vi "process_reaction_methodr.vi"() -> ()   [LabVIEW 2021]
uses:
  <vilib>/Analysis/NI_AALPro.lvlib
panel:
  out "appended array":dbl[][](array[numeric])=[[0.0, 0.0], [0.4, 0.01], [0.8, 0.07], [1.2, 0.17], [1.6, 0.31], [2.0, 0.46], [2.4, 0.62], [2.8, 0.76], [3.2, 0.88], [3.6, 0.99], [4.0, 1.09], [4.4, 1.16], [4.8, 1.22], [5.2, 1.27], [5.6, 1.31], [6.0, 1.34], [6.4, 1.36], [6.8, 1.38], [7.2, 1.39], [7.6, 1.4], [8.0, 1.412], [8.4, 1.41], [8.8, 1.427], [9.6, 1.42], [10.0, 1.42]]
  in  "Values for output y":dbl[](array[numeric])=[0.0, 0.01, 0.07, 0.17, 0.31, 0.46, 0.62, 0.76, 0.88, 0.99, 1.09, 1.16, 1.22, 1.27, 1.31, 1.34, 1.36, 1.38, 1.39, 1.4, 1.412, 1.41, 1.427, 1.42, 1.42]
  in  "values for time t":dbl[](array[numeric])=[0.0, 0.4, 0.8, 1.2, 1.6, 2.0, 2.4, 2.8, 3.2, 3.6, 4.0, 4.4, 4.8, 5.2, 5.6, 6.0, 6.4, 6.8, 7.2, 7.6, 8.0, 8.4, 8.8, 9.6, 10.0]
  out "L":dbl=0.8000000000000003
  out "T":dbl=3.664516129032257
  out "K":dbl=1.42
  out "max index(es)":i32=5
  out "max dy/dt":dbl=0.38750000000000007
  out "output array 2":dbl[](array[numeric])=[0.0, 0.4, 0.8, 1.2, 1.6, 2.0, 2.4, 2.8, 3.2, 3.6, 4.0, 4.4, 4.8, 5.2, 5.6, 6.0, 6.4, 6.8, 7.2, 7.6, 8.0, 8.4, 8.8, 9.6, 10.0]
  out "output array":dbl[](array[numeric])=[0.0, 0.01, 0.07, 0.17, 0.31, 0.46, 0.62, 0.76, 0.88, 0.99, 1.09, 1.16, 1.22, 1.27, 1.31, 1.34, 1.36, 1.38, 1.39, 1.4, 1.412, 1.41, 1.427, 1.42, 1.42]
  in  "U":dbl=1.0
  out "Delta_Y":dbl=1.42
  out "size(s)":i32[](array[numeric])=[25, 2]
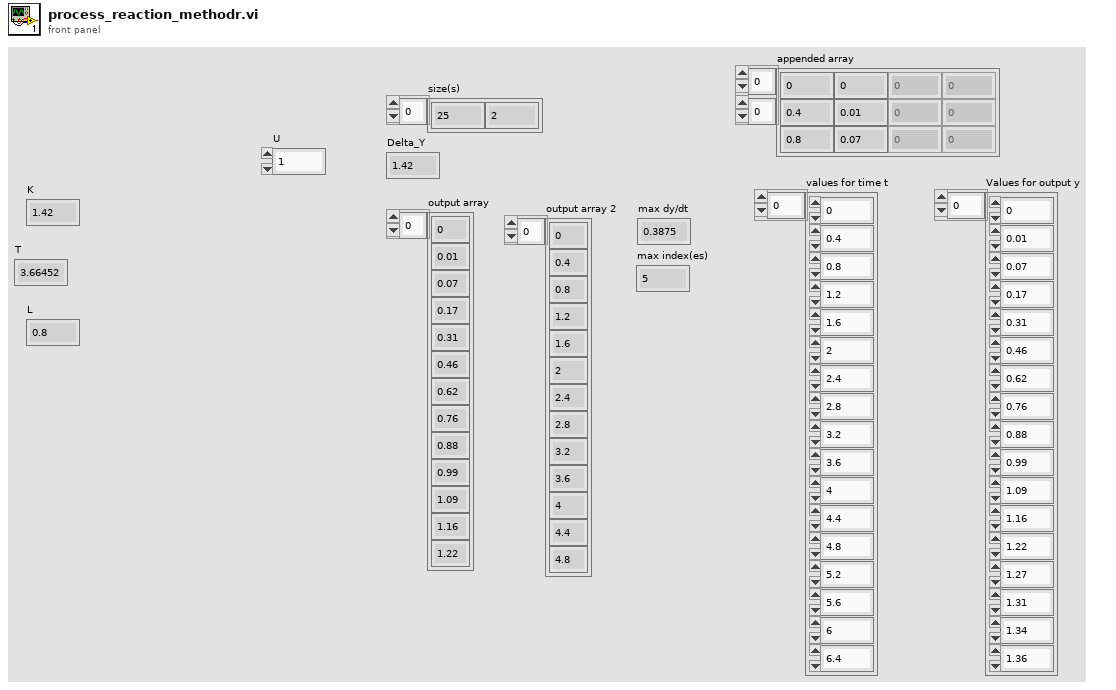
[diagram p1: front panel]
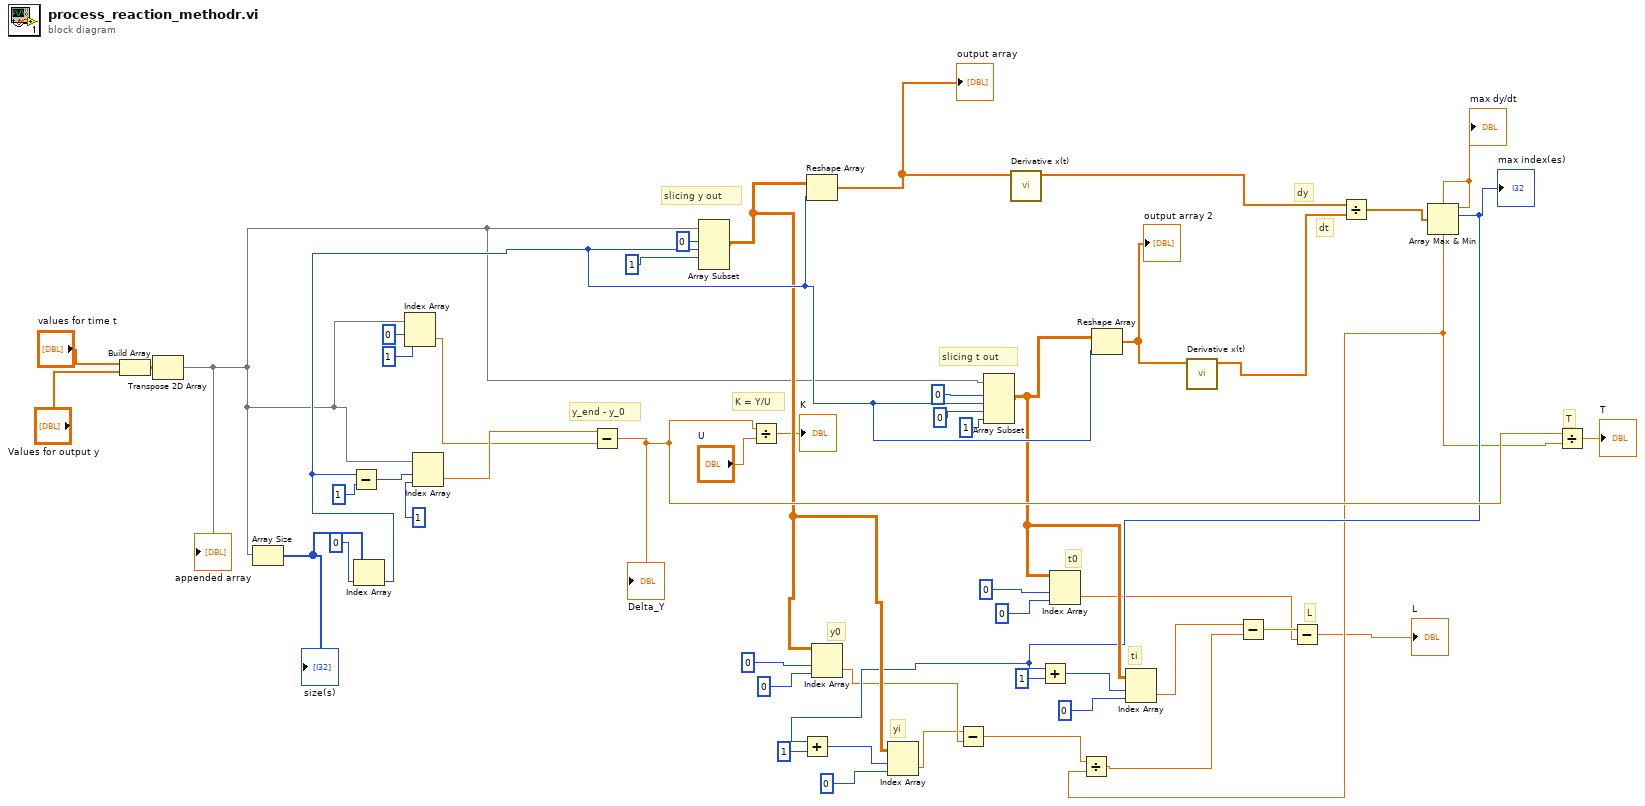
[diagram p0: block diagram]
diagram:
  # "L"
  # "yi"
  # "y0"
  # "ti"
  # "t0"
  # "T"
  # "dt"
  # "dy"
  # "slicing t out"
  # "slicing y out"
  # "K = Y/U"
  # "y_end - y_0"
  n1 = Build Array("values for time t", "Values for output y") -> (w2:dbl[][])
  n2 = Transpose 2D Array(2D array=w2) -> (transposed array=w1:dbl[][])
  "appended array" <- w1
  n3 = Array Size(array=w1) -> (size(s)=w45:i32[])
  "size(s)" <- w45
  n4 = Index Array(array=w45, index=0) -> (element=w34:i32)
  n5 = Subtract(x=w34, y=1) -> (x-y=w42:i32)
  n6 = Index Array(array=w1, index (row)=0 ("index"), index (col)=1 ("disabled index (col)")) -> (element=w48:dbl)
  n7 = Index Array(array=w1, index (row)=w42, index (col)=1 ("disabled index (col)")) -> (element=w50:dbl)
  n8 = Subtract(x=w50, y=w48) -> (x-y=w29:dbl)
  "Delta_Y" <- w29
  n9 = Array Subset(array=w1, index (row)=0 ("index"), length (row)=w34, index (col)=1 ("index")) -> (w17:dbl[][])  [unwired: 1 in]
  n10 = Divide(x=w29, y="U") -> (x/y=→"K":dbl)
  n11 = Reshape Array(w17, w34) -> (w39:dbl[])
  "output array" <- w39
  n12 = Index Array(array=w17, index (row)=0, index (col)=0 ("disabled index (col)")) -> (element=w15:dbl)
  n13 = Array Subset(array=w1, index (row)=0 ("index"), length (row)=w34, index (col)=0 ("index"), length (col)=1 ("length")) -> (w23:dbl[][])
  n14 = call <vilib>:"Derivative x(t).vi"("X"=w39) -> ("dX/dt"=w32:dbl[])  [unwired: 9 in, 1 out]
  n15 = Index Array(array=w23, index (row)=0, index (col)=0 ("disabled index (col)")) -> (element=w8:dbl)
  n16 = Reshape Array(w23, w34) -> (w37:dbl[])
  "output array 2" <- w37
  n17 = call <vilib>:"Derivative x(t).vi"("X"=w37) -> ("dX/dt"=w31:dbl[])  [unwired: 9 in, 1 out]
  n18 = Divide(x=w32, y=w31) -> (x/y=w30:dbl[])
  n19 = Array Max & Min(array=w30) -> (max value=w12:dbl, max index (indices)=w16:i32)  [unwired: 2 out]
  "max dy/dt" <- w12
  "max index(es)" <- w16
  n20 = Add(x=w16, y=1) -> (x+y=w18:i32)
  n21 = Index Array(array=w17, index (row)=w18, index (col)=0 ("disabled index (col)")) -> (element=w14:dbl)
  n22 = Subtract(x=w14, y=w15) -> (x-y=w13:dbl)
  n23 = Add(x=w16, y=1) -> (x+y=w24:i32)
  n24 = Divide(x=w13, y=w12) -> (x/y=w10:dbl)
  n25 = Index Array(array=w23, index (row)=w24, index (col)=0 ("disabled index (col)")) -> (element=w11:dbl)
  n26 = Subtract(x=w11, y=w10) -> (x-y=w9:dbl)
  n27 = Subtract(x=w9, y=w8) -> (x-y=→"L":dbl)
  n28 = Divide(x=w29, y=w12) -> (x/y=→"T":dbl)
